vi "ZeroAxis.vi"(8 "error in (no error)":errorcluster, 10 "Axis":T1, 11 "MotorController in":refnum<class "MotorController.lvclass">) -> (0 "error out":errorcluster, 3 "MotorController out":refnum<class "MotorController.lvclass">)   [LabVIEW 2019, in "MotorController.lvclass"]
uses:
  MotorController.lvclass
  Axes_enum_typedef.ctl
  MotorController.lvclass/MotorController.ctl
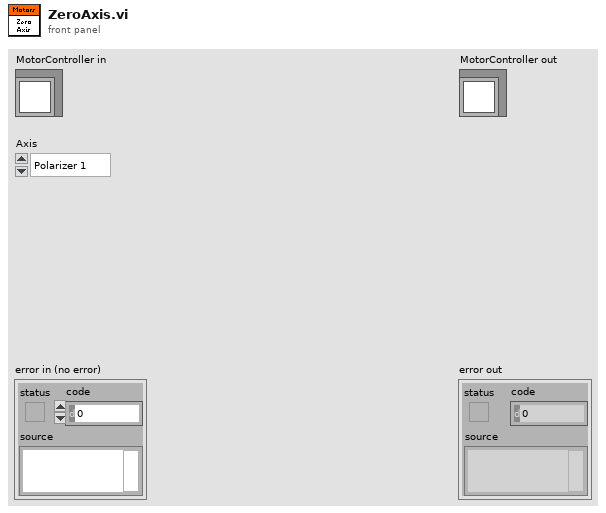
[diagram p1: front panel]
types:
  T1 = typedef "Axes_enum_typedef.ctl" = enum16{"Polarizer 1", "Polarizer 2", "Sample", "Stage"}
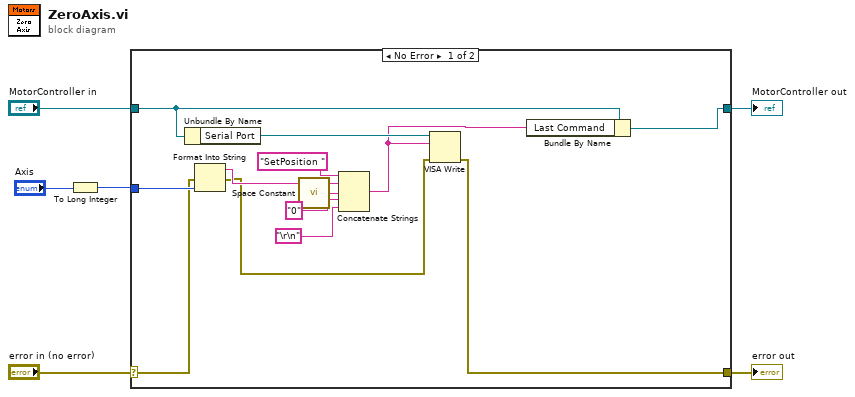
[diagram p0: block diagram]
diagram:
  n1 = To Long Integer(number="Axis") -> (32bit integer=w2:i32)
  n2 = case shown="No Error" "error in (no error)" {
    selector: "error in (no error)" -> [w17 w21]
    tunnel: [w10 w21] -> w5
    tunnel: [w7 w20] -> w3
    tunnel: "MotorController in" -> [w9 w20]
    tunnel: w2 -> [w18 _]
    frame No Error {
      n3 = Unbundle By Name(w9) -> ("Serial Port"=w12:refnum<visa-resource-name>)
      n4 = Format Into String(error in=w17, w18) -> (resulting string=w16:string, error out=w11:errorcluster)  [unwired: 2 in]
      n5 = call <vilib>:"Space Constant.vi"() -> ("String"=w15:string)
      n6 = Concatenate Strings("SetPosition " ("string"), w16, w15, "0" ("string"), "\r\n") -> (w8:string)
      n7 = VISA Write(VISA resource name=w12, write buffer=w8, error in (no error)=w11) -> (error out=w10:errorcluster)  [unwired: 2 out]
      n8 = Bundle By Name(cluster=w9, "Last Command"=w8) -> (w7:refnum<class "MotorController.lvclass">)
    }
    frame Error {
    }
  }
  "error out" <- w5
  "MotorController out" <- w3
